vi "GEOM_AmpsizeVariable2numbers.vi"(7 "separator":string=",", 9 "detrows":i32, 10 "detcols":i32, 11 "ampval":string) -> (1 "amprows":i32, 2 "ampcols":i32)   [LabVIEW 2016]
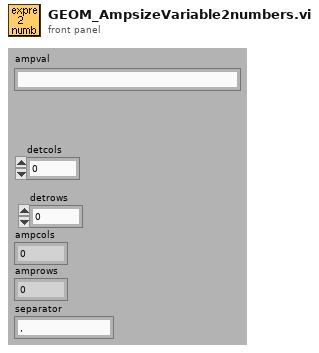
[diagram p1: front panel]
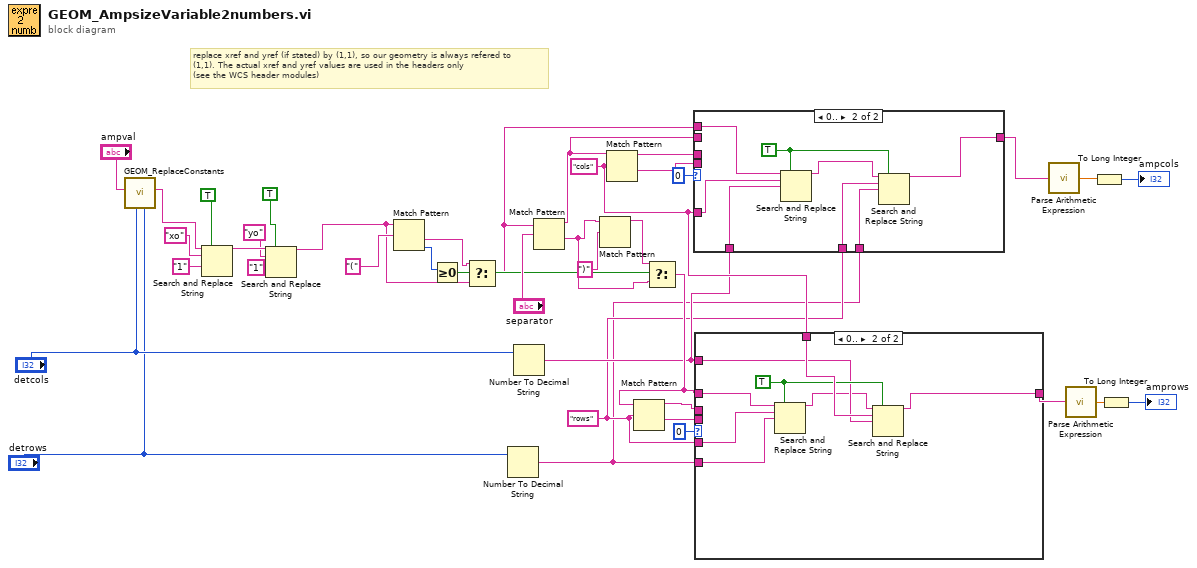
[diagram p0: block diagram]
diagram:
  w16 = "rows" ("regular expression")
  w18 = "cols" ("regular expression")
  # "replace xref and yref (if stated) by (1,1), so our geometry is always refered to\n(1,1). The actual xref and yref values are used in the headers only\n(see the WCS header modules)"
  n1 = call "GEOM_ReplaceConstants.vi"("detrows"="detrows", "detcols"="detcols", "ampval"="ampval") -> ("ampval out"=w5:string)  [unwired: 8 out]
  n2 = Search and Replace String(replace all?=TRUE ("replace all? (F)"), input string=w5, search string="xo", replace string="1" ("replace string (\"\")")) -> (result string=w11:string)  [unwired: 1 in, 6 out]
  n3 = Search and Replace String(replace all?=TRUE ("replace all? (F)"), input string=w11, search string="yo", replace string="1" ("replace string (\"\")")) -> (result string=w7:string)  [unwired: 1 in, 6 out]
  n4 = Match Pattern(string=w7, regular expression="(") -> (after substring=w24:string, offset past match=w25:i32)  [unwired: 3 out]
  n5 = Greater Or Equal To 0?(x=w25) -> (x >= 0?=w23:bool)
  n6 = Select(t=w24, s=w23, f=w7) -> (s? t:f=w19:string)
  n7 = Number To Decimal String(number="detrows") -> (decimal integer string=w15:string)  [unwired: 1 out]
  n8 = Number To Decimal String(number="detcols") -> (decimal integer string=w17:string)  [unwired: 1 out]
  n9 = Match Pattern(string=w19, regular expression="separator") -> (before substring=w34:string, after substring=w21:string)  [unwired: 3 out]
  n10 = Match Pattern(string=w21, regular expression=")") -> (before substring=w22:string)  [unwired: 4 out]
  n11 = Match Pattern(string=w34, regular expression=w18) -> (before substring=w31:string, after substring=w30:string)  [unwired: 3 out]
  n12 = Select(t=w22, s=w23, f=w21) -> (s? t:f=w20:string)
  n13 = Match Pattern(string=w20, regular expression=w16) -> (before substring=w27:string, after substring=w26:string)  [unwired: 3 out]
  n14 = case shown="0.." 0 ("offset past match") {
    tunnel: w34 -> [w40 _]
    tunnel: [w40 w41] -> w33
    tunnel: w31 -> [_ _]
    tunnel: w30 -> [_ _]
    tunnel: w19 -> [_ w46]
    tunnel: w18 -> [_ w45]
    tunnel: w17 -> [_ w44]
    tunnel: w16 -> [_ w43]
    tunnel: w15 -> [_ w42]
    frame Default {
    }
    frame 0.. {
      w48 = TRUE ("replace all? (F)")
      n15 = Search and Replace String(replace all?=w48, input string=w46, search string=w45, replace string=w44) -> (result string=w47:string)  [unwired: 1 in, 6 out]
      n16 = Search and Replace String(replace all?=w48, input string=w47, search string=w43, replace string=w42) -> (result string=w41:string)  [unwired: 1 in, 6 out]
    }
  }
  n17 = case shown="0.." 0 ("offset past match") {
    tunnel: w20 -> [w49 w57]
    tunnel: [w49 w50] -> w29
    tunnel: w27 -> [_ _]
    tunnel: w26 -> [_ _]
    tunnel: w16 -> [_ w56]
    tunnel: w18 -> [_ w55]
    tunnel: w15 -> [_ w53]
    tunnel: w17 -> [_ w52]
    frame Default {
    }
    frame 0.. {
      w54 = TRUE ("replace all? (F)")
      n18 = Search and Replace String(replace all?=w54, input string=w57, search string=w56, replace string=w53) -> (result string=w51:string)  [unwired: 1 in, 6 out]
      n19 = Search and Replace String(replace all?=w54, input string=w51, search string=w55, replace string=w52) -> (result string=w50:string)  [unwired: 1 in, 6 out]
    }
  }
  n20 = call "Parse Arithmetic Expression.vi"("Arithmetic Expression"=w33) -> ("Result"=w32:dbl)
  n21 = call "Parse Arithmetic Expression.vi"("Arithmetic Expression"=w29) -> ("Result"=w28:dbl)
  n22 = To Long Integer(number=w32) -> (32bit integer=→"ampcols":i32)
  n23 = To Long Integer(number=w28) -> (32bit integer=→"amprows":i32)
